vi "Read Average.vi"(8 "error in (no error)":errorcluster, 11 "Averager in":refnum<class "Averager.lvclass">) -> (0 "error out":errorcluster, 2 "Average":dbl, 3 "Averager out":refnum<class "Averager.lvclass">)   [LabVIEW 2018, in "Averager.lvclass"]
uses:
  Averager.lvclass
  Averager.lvclass/Averager.ctl
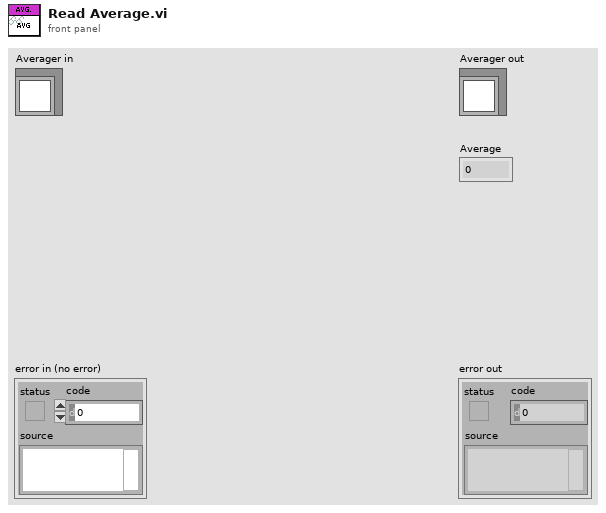
[diagram p1: front panel]
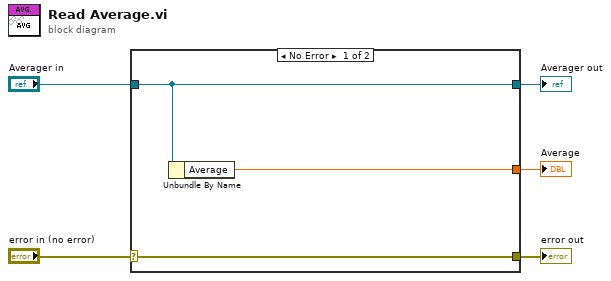
[diagram p0: block diagram]
diagram:
  n1 = case shown="No Error" "error in (no error)" {
    selector: "error in (no error)" -> [w8 w9]
    tunnel: [w8 w9] -> w4
    tunnel: [w7 w10] -> w2
    tunnel: "Averager in" -> [w7 w10]
    tunnel: [w6 _] -> w1
    frame No Error {
      n2 = Unbundle By Name(w7) -> ("Average"=w6:dbl)
    }
    frame Error {
    }
  }
  "error out" <- w4
  "Averager out" <- w2
  "Average" <- w1
